vi "SwerveModuleReadData.vi"(8 "Swerve Disable":bool, 10 "NT Name (Errors)":string, 11 "NT Name (Details)":string) -> (0 "Shifter State":string, 1 "Drive Velocity":dbl format="%.1f", 2 "Drive Temperature":dbl, 3 "Azimuth Position":dbl format="%.1f", 4 "Shifter Failure":T1, 5 "Drive Overheating":T1, 6 "Drive Fault":T1, 7 "Azimuth Fault":T1)   [LabVIEW 2023]
uses:
  <vilib>/Rock Robotics/Network Tables/NT Read Numeric Array.vi
  <vilib>/Rock Robotics/Network Tables/NT Read Boolean Array.vi
  GlobalDashboard.vi
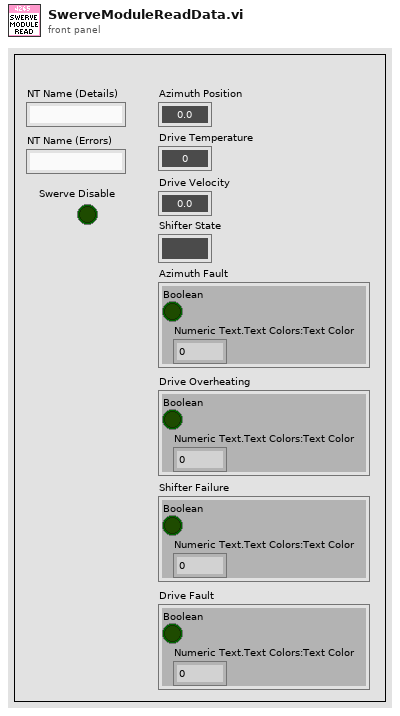
[diagram p1: front panel]
types:
  T1 = cluster{"Boolean":bool, "Numeric Text.Text Colors:Text Color":u32}
  T2 = cluster{bool, "Numeric Text.Text Colors:Text Color":u32}
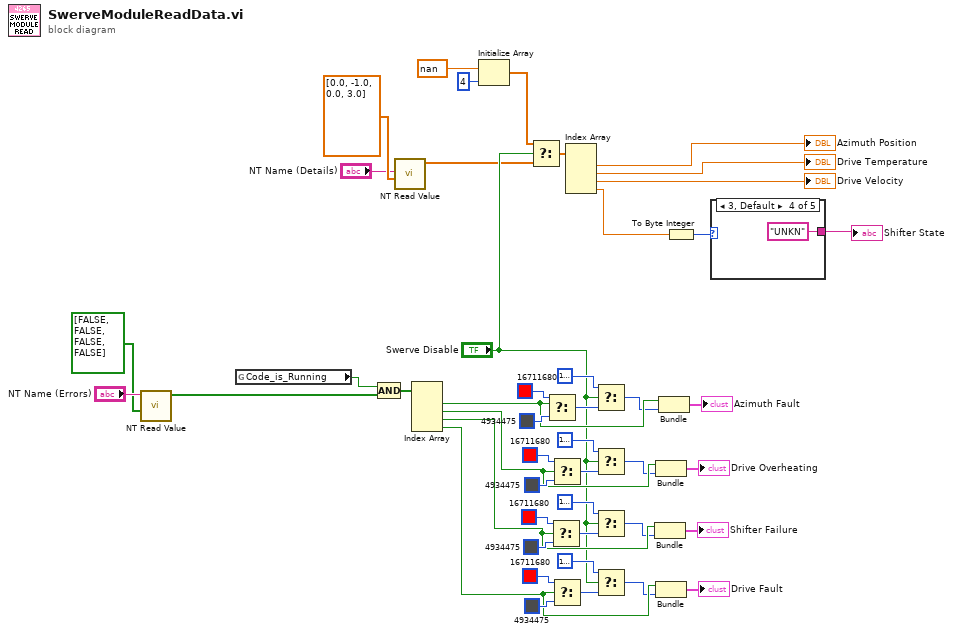
[diagram p0: block diagram]
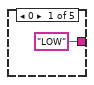
[diagram p2: hidden frame]
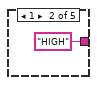
[diagram p3: hidden frame]
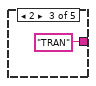
[diagram p4: hidden frame]
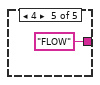
[diagram p5: hidden frame]
diagram:
  n1 = call-poly <vilib>:"NT Read Value.vi"("default value"=bool[] [FALSE, FALSE, FALSE, FALSE], "name"="NT Name (Errors)") -> ("value"=w43:bool[])  [unwired: 7 in, 2 out]
  n2 = global read "GlobalDashboard.vi" "Code_is_Running"() -> (w28:bool)
  n3 = Compound Arithmetic op=AND(w28, w43) -> (w29:bool[])
  n4 = call-poly <vilib>:"NT Read Value.vi"("default value"=dbl[] [0.0, -1.0, 0.0, 3.0] ("Default Value"), "name"="NT Name (Details)") -> ("value"=w1:dbl[])  [unwired: 7 in, 2 out]
  n5 = Index Array(array=w29) -> (element #1=w40:bool, element #2=w32:bool, element #3=w24:bool, element #4=w23:bool)  [unwired: 4 in]
  n6 = Initialize Array(nan, 4 ("dimension size")) -> (w8:dbl[])
  n7 = Select(t=w8, s="Swerve Disable", f=w1) -> (s? t:f=w6:dbl[])
  n8 = Select(t=u32 16711680 ("Numeric Text.Text Colors:Text Color"), s=w40, f=u32 4934475 ("Numeric Text.Text Colors:Text Color")) -> (s? t:f=w22:u32)
  n9 = Select(t=u32 16711680 ("Numeric Text.Text Colors:Text Color"), s=w24, f=u32 4934475 ("Numeric Text.Text Colors:Text Color")) -> (s? t:f=w16:u32)
  n10 = Select(t=u32 16711680 ("Numeric Text.Text Colors:Text Color"), s=w32, f=u32 4934475 ("Numeric Text.Text Colors:Text Color")) -> (s? t:f=w18:u32)
  n11 = Select(t=u32 16711680 ("Numeric Text.Text Colors:Text Color"), s=w23, f=u32 4934475 ("Numeric Text.Text Colors:Text Color")) -> (s? t:f=w14:u32)
  n12 = Index Array(array=w6) -> (element #1=→"Azimuth Position":dbl, element #2=→"Drive Temperature":dbl, element #3=→"Drive Velocity":dbl, element #4=w2:dbl)  [unwired: 4 in]
  n13 = Select(t=u32 16777222 ("Numeric Text.Text Colors:Text Color"), s="Swerve Disable", f=w22) -> (s? t:f=w20:u32)
  n14 = Select(t=u32 16777222 ("Numeric Text.Text Colors:Text Color"), s="Swerve Disable", f=w18) -> (s? t:f=w13:u32)
  n15 = Select(t=u32 16777222 ("Numeric Text.Text Colors:Text Color"), s="Swerve Disable", f=w16) -> (s? t:f=w12:u32)
  n16 = Select(t=u32 16777222 ("Numeric Text.Text Colors:Text Color"), s="Swerve Disable", f=w14) -> (s? t:f=w11:u32)
  n17 = Bundle(w24, "Numeric Text.Text Colors:Text Color"=w12) -> (→"Shifter Failure":T2)  [unwired: 1 in]
  n18 = Bundle(w32, "Numeric Text.Text Colors:Text Color"=w13) -> (→"Drive Overheating":T2)  [unwired: 1 in]
  n19 = Bundle(w23, "Numeric Text.Text Colors:Text Color"=w11) -> (→"Drive Fault":T2)  [unwired: 1 in]
  n20 = Bundle(w40, "Numeric Text.Text Colors:Text Color"=w20) -> (→"Azimuth Fault":T2)  [unwired: 1 in]
  n21 = To Byte Integer(number=w2) -> (8bit integer=w44:i8)
  n22 = case shown="3, Default" w44 {
    tunnel: ["LOW" "HIGH" "TRAN" "UNKN" "FLOW"] -> w45
    frame 0 {
    }
    frame 1 {
    }
    frame 2 {
    }
    frame 3, Default {
    }
    frame 4 {
    }
  }
  "Shifter State" <- w45
